vi "LINC ID Global.vi"(5 "target name":string, 7 "mode":T1, 8 "error in (no error)":errorcluster, 11 "type (CMD)":enum16{"CMD", "TLM"}(ring)) -> (0 "error out":errorcluster, 2 "ID":i32)   [LabVIEW 2018, in "STEPkgDriver_LINC.lvlib"]
uses:
  STEPkgDriver_LINC.lvlib
  LINC Global ID Mode.ctl
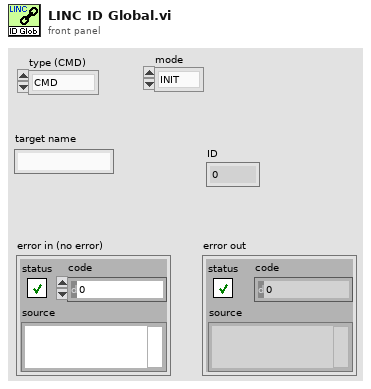
[diagram p1: front panel]
types:
  T1 = typedef "STEPkgDriver_LINC.lvlib/LINC Global ID Mode.ctl" = enum16{"INIT", "CLEAR", "GET_ID"}
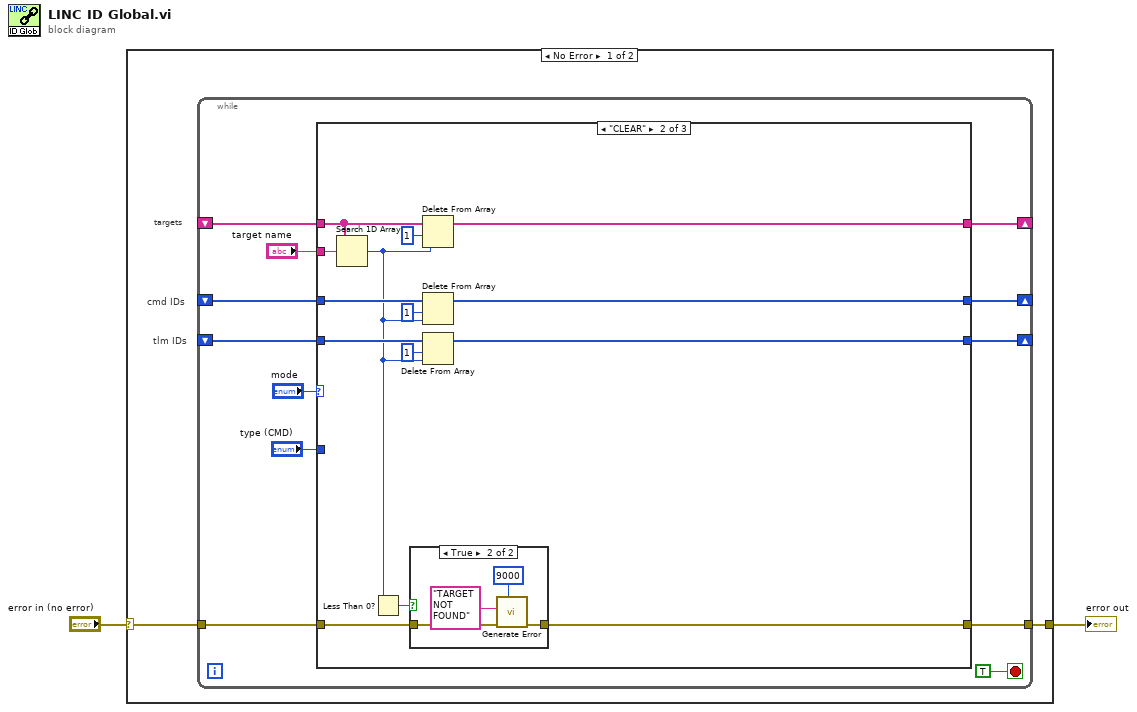
[diagram p0: block diagram]
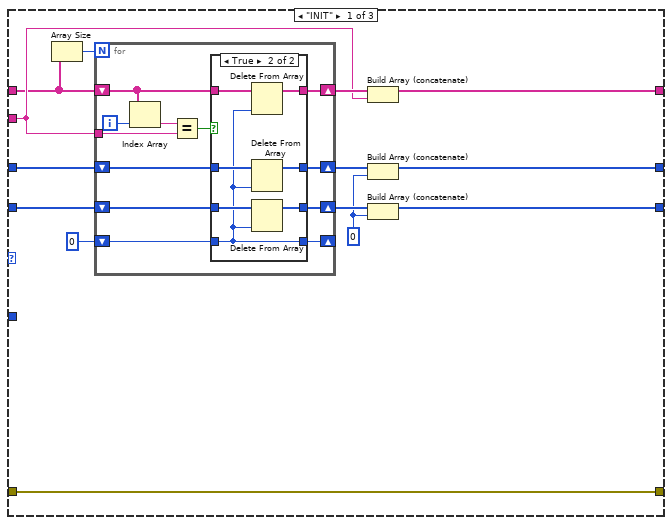
[diagram p2: hidden frame]
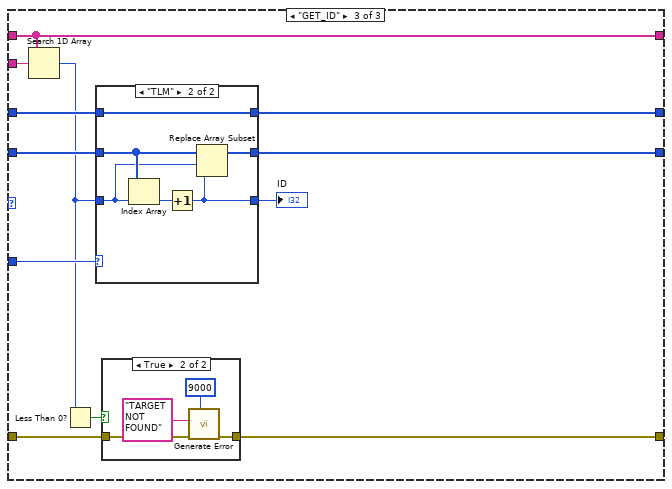
[diagram p5: hidden frame]
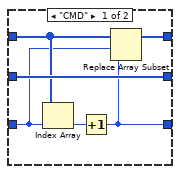
[diagram p6: hidden frame]
diagram:
  n1 = case shown="No Error" "error in (no error)" {
    selector: "error in (no error)" -> [w4 w103]
    tunnel: [w3 w103] -> w1
    frame No Error {
      # "tlm IDs"
      # "cmd IDs"
      # "targets"
      n2 = while {
        shift-right: [w12] -> _
        shift-left: _ -> [w14]
        shift-right: [w9] -> _
        shift-left: _ -> [w11]
        shift-right: [w8] -> _
        shift-left: _ -> [w10]
        tunnel: w4 -> [w7]
        tunnel: [w6] -> w3
        stop <- TRUE stop-if-true
        n3 = case shown="\"CLEAR\"" "mode" {
          tunnel: w14 -> [w18 w64 w82]
          tunnel: "target name" -> [w26 w55 w81]
          tunnel: [w25 w63 w82] -> w12
          tunnel: w11 -> [w19 w62 w79]
          tunnel: w10 -> [w29 w61 w78]
          tunnel: [w23 w60 w76] -> w9
          tunnel: [w21 w59 w77] -> w8
          tunnel: w7 -> [w17 w58 w84]
          tunnel: [w17 w56 w83] -> w6
          tunnel: "type (CMD)" -> [_ _ w80]
          frame "INIT" {
            w20 = 0
            n4 = Array Size(array=w18) -> (size(s)=w30:i32)
            n5 = for {
              N: w30 -> [_]
              shift-right: [w35] -> w27
              shift-left: w18 -> [w41]
              shift-right: [w34] -> w24
              shift-left: w19 -> [w40]
              shift-right: [w33] -> w22
              shift-left: w29 -> [w39]
              tunnel: w26 -> [w37]
              shift-right: [w31] -> _
              shift-left: 0 -> [w32]
              i -> [w42]
              n6 = Index Array(array=w41, index=w42) -> (element=w38:string)
              n7 = Equal?(x=w38, y=w37) -> (x = y?=w36:bool)
              n8 = case shown="True" w36 {
                tunnel: w41 -> [w47 w54]
                tunnel: w40 -> [w46 w52]
                tunnel: w39 -> [w45 w51]
                tunnel: [w47 w53] -> w35
                tunnel: [w46 w50] -> w34
                tunnel: [w45 w49] -> w33
                tunnel: w32 -> [w44 w48]
                tunnel: [w43 w48] -> w31
                frame False {
                  n9 = Increment(x=w44) -> (x+1=w43:i32)
                }
                frame True {
                  n10 = Delete From Array(array=w54, index=w48) -> (array with subset deleted=w53:string[])  [unwired: 1 in, 1 out]
                  n11 = Delete From Array(array=w52, index=w48) -> (array with subset deleted=w50:i32[])  [unwired: 1 in, 1 out]
                  n12 = Delete From Array(array=w51, index=w48) -> (array with subset deleted=w49:i32[])  [unwired: 1 in, 1 out]
                }
              }
            }
            n13 = Build Array (concatenate)(w27, w26) -> (w25:string[])
            n14 = Build Array (concatenate)(w24, w20) -> (w23:i32[])
            n15 = Build Array (concatenate)(w22, w20) -> (w21:i32[])
          }
          frame "CLEAR" {
            n16 = Search 1D Array(1D array=w64, element=w55) -> (index of element=w57:i32)  [unwired: 1 in]
            n17 = Less Than 0?(x=w57) -> (x < 0?=w67:bool)
            n18 = case shown="True" w67 {
              tunnel: w58 -> [w69 w73]
              tunnel: [w69 w72] -> w56
              frame False {
              }
              frame True {
                n19 = call "Generate Error.vi"("error code (-1301)"=9000, "error in"=w73, "description"="TARGET NOT FOUND") -> ("error out"=w72:errorcluster)  [unwired: 8 in]
              }
            }
            n20 = Delete From Array(array=w64, length=1, index=w57) -> (array with subset deleted=w63:string[])  [unwired: 1 out]
            n21 = Delete From Array(array=w62, length=1, index=w57) -> (array with subset deleted=w60:i32[])  [unwired: 1 out]
            n22 = Delete From Array(array=w61, length=1, index=w57) -> (array with subset deleted=w59:i32[])  [unwired: 1 out]
          }
          frame "GET_ID" {
            n23 = Search 1D Array(1D array=w82, element=w81) -> (index of element=w75:i32)  [unwired: 1 in]
            n24 = Less Than 0?(x=w75) -> (x < 0?=w85:bool)
            n25 = case shown="\"TLM\"" w80 {
              tunnel: w79 -> [w90 w97]
              tunnel: w78 -> [w91 w95]
              tunnel: [w91 w94] -> w77
              tunnel: [w89 w97] -> w76
              tunnel: w75 -> [w88 w93]
              tunnel: [w86 w92] -> w74
              frame "CMD" {
                n26 = Index Array(array=w90, index=w88) -> (element=w87:i32)
                n27 = Increment(x=w87) -> (x+1=w86:i32)
                n28 = Replace Array Subset(array=w90, new element=w86, index=w88) -> (w89:i32[])
              }
              frame "TLM" {
                n29 = Index Array(array=w95, index=w93) -> (element=w96:i32)
                n30 = Increment(x=w96) -> (x+1=w92:i32)
                n31 = Replace Array Subset(array=w95, new element=w92, index=w93) -> (w94:i32[])
              }
            }
            "ID" <- w74
            n32 = case shown="True" w85 {
              tunnel: w84 -> [w98 w102]
              tunnel: [w98 w101] -> w83
              frame False {
              }
              frame True {
                n33 = call "Generate Error.vi"("error code (-1301)"=9000, "error in"=w102, "description"="TARGET NOT FOUND") -> ("error out"=w101:errorcluster)  [unwired: 8 in]
              }
            }
          }
        }
      }
    }
    frame Error {
    }
  }
  "error out" <- w1
